vi "GetItemByPath.vi"(8 "error in (no error)":errorcluster, 9 "Path":string, 10 "Remove?":bool, 11 "CDependencyList in":refnum<class "CDependencyList.lvclass">) -> (0 "error out":errorcluster, 1 "ILabVIEWItem":refnum<class "ILabVIEWItem.lvclass">, 2 "key found?":bool, 3 "CDependencyList out":refnum<class "CDependencyList.lvclass">)   [LabVIEW 2020, in "DependencyInspection.lvlib" / "CDependencyList.lvclass"]
uses:
  CDependencyList.lvclass
  LabVIEWObjectInterfaces/ILabVIEWItem/ILabVIEWItem.lvclass
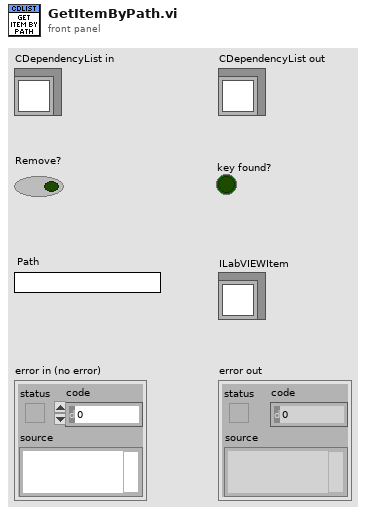
[diagram p1: front panel]
types:
  T1 = typedef "DependencyInspection.lvlib/CDependencyList.lvclass/DependencyListRef.ctl" = refnum<data-value>
  T2 = typedef "DependencyInspection.lvlib/CDependencyList.lvclass/DependencyList.ctl" = map{string, refnum<class "ILabVIEWItem.lvclass">}
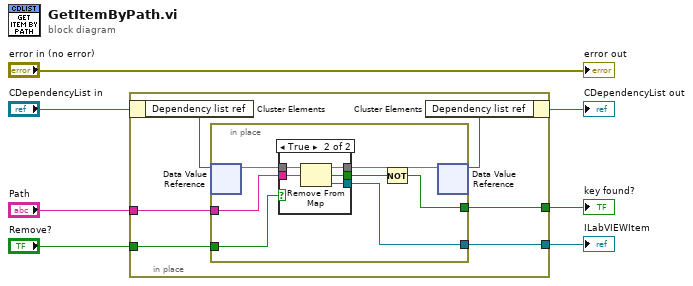
[diagram p0: block diagram]
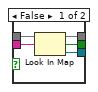
[diagram p2: hidden frame]
diagram:
  n1 = in-place {
    in-place-border: "Path" -> [w13]
    in-place-border: [w12] -> w5
    in-place-border: [w11] -> w4
    in-place-border: "Remove?" -> [w8]
    n2 = in-place-cluster #1("CDependencyList in") -> ("Dependency list ref"=w10:T1)
    n3 = in-place {
      in-place-border: w13 -> [w20]
      in-place-border: [w19] -> w12
      in-place-border: [w18] -> w11
      in-place-border: w8 -> [w15]
      n4 = in-place-dvr #2(w10) -> (w16:T2)  [unwired: 1 out]
      n5 = case shown="True" w15 {
        tunnel: w20 -> [w24 w27]
        tunnel: [w23 w25] -> w18
        tunnel: [w22 w26] -> w17
        tunnel: w16 -> [w21 w29]
        tunnel: [w21 w28] -> w14
        frame False {
          n6 = Look In Map(map=w21, key=w24) -> (key not found?=w22:bool, value=w23:refnum<class "ILabVIEWItem.lvclass">)  [unwired: 1 in]
        }
        frame True {
          n7 = Remove From Map(10:w27, 11:w29) -> (1:w25:refnum<class "ILabVIEWItem.lvclass">, 2:w26:bool, 3:w28:T2)
        }
      }
      n8 = Not(x=w17) -> (.not. x?=w19:bool)
      n9 = in-place-dvr #2(w14) -> (w9:T1)  [unwired: 1 out]
    }
    n10 = in-place-cluster #1("Dependency list ref"=w9) -> (→"CDependencyList out":refnum<class "CDependencyList.lvclass">)
  }
  "key found?" <- w5
  "ILabVIEWItem" <- w4
  "error out" <- "error in (no error)"
